vi "Initialize.vi"(8 "error in (no error)":errorcluster, 11 "AG in":refnum<class "AG.lvclass">) -> (0 "error out":errorcluster, 3 "AG out":refnum<class "AG.lvclass">)   [LabVIEW 2018, in "AG.lvclass"]
uses:
  AG.lvclass
  AG.lvclass/AG.ctl
  Client/Client.lvclass
  Comm/Stream/Stream.lvclass
  Log/Log.lvclass
  Device/angles/angles.lvclass
  StateMachine/State Machine.lvclass
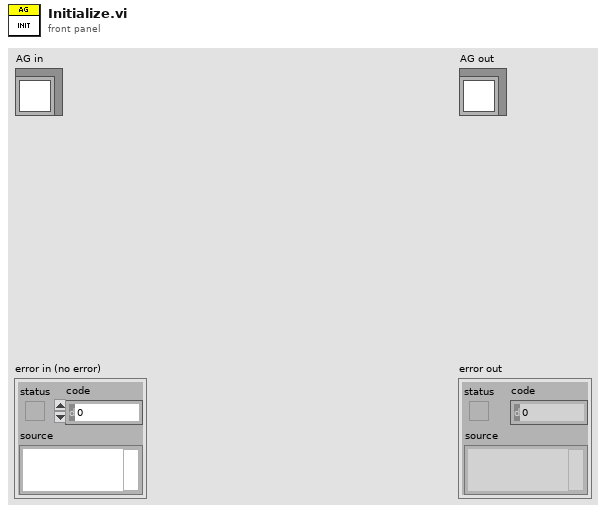
[diagram p1: front panel]
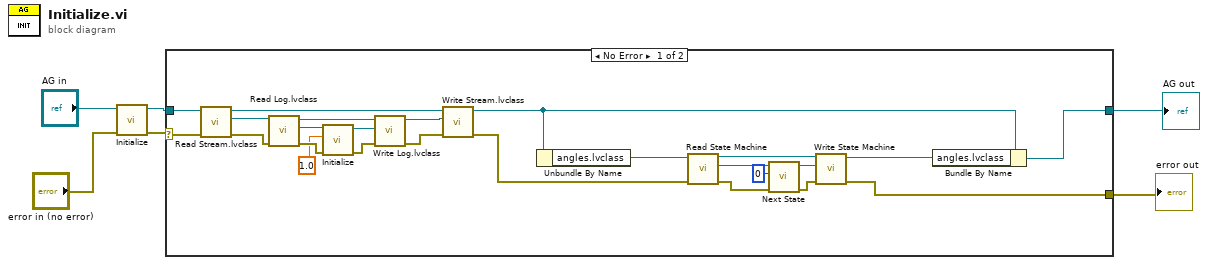
[diagram p0: block diagram]
diagram:
  n1 = call-parent "Initialize.vi"("error in (no error)"="error in (no error)", "Client in"="AG in") -> ("error out"=w3:errorcluster, "Client out"=w4:refnum<class "AG.lvclass">)  [unwired: 8 in]
  n2 = case shown="No Error" w3 {
    selector: w3 -> [w9 w33]
    tunnel: [w23 w32] -> w1
    tunnel: w4 -> [w10 w32]
    tunnel: [w11 w33] -> w2
    frame No Error {
      n3 = call-dynamic "Read Stream.lvclass.vi"("error in (no error)"=w9, "Client in"=w10) -> ("error out"=w7:errorcluster, "Stream.lvclass"=w8:refnum<class "Stream.lvclass">, "Client out"=w31:refnum<class "AG.lvclass">)  [unwired: 7 in]
      n4 = call-dynamic "Read Log.lvclass.vi"("error in (no error)"=w7, "Comm in"=w8) -> ("error out"=w19:errorcluster, "Log.lvclass"=w21:refnum<class "Log.lvclass">, "Comm out"=w22:refnum<class "Stream.lvclass">)  [unwired: 7 in]
      n5 = call-dynamic "Initialize.vi"("error in (no error)"=w19, "Level"=1.0, "Log in"=w21) -> ("error out"=w18:errorcluster, "Log out"=w20:refnum<class "Log.lvclass">)  [unwired: 7 in]
      n6 = call-dynamic "Write Log.lvclass.vi"("error in (no error)"=w18, "Log.lvclass"=w20, "Comm in"=w22) -> ("error out"=w16:errorcluster, "Comm out"=w17:refnum<class "Stream.lvclass">)  [unwired: 7 in]
      n7 = call-dynamic "Write Stream.lvclass.vi"("error in (no error)"=w16, "Stream.lvclass"=w17, "Client in"=w31) -> ("error out"=w13:errorcluster, "Client out"=w24:refnum<class "AG.lvclass">)  [unwired: 7 in]
      n8 = Unbundle By Name(w24) -> ("angles.lvclass"=w14:refnum<class "angles.lvclass">)
      n9 = call-dynamic "Read State Machine.vi"("error in (no error)"=w13, "Device in"=w14) -> ("error out"=w27:errorcluster, "State Machine.lvclass"=w30:refnum<class "State Machine.lvclass">, "Device out"=w29:refnum<class "angles.lvclass">)  [unwired: 7 in]
      n10 = call "Next State.vi"("error in (no error)"=w27, "New_State"=0, "State Machine in"=w30) -> ("error out"=w26:errorcluster, "State Machine out"=w28:refnum<class "State Machine.lvclass">)  [unwired: 7 in]
      n11 = call-dynamic "Write State Machine.vi"("error in (no error)"=w26, "State Machine.lvclass"=w28, "Device in"=w29) -> ("error out"=w11:errorcluster, "Device out"=w25:refnum<class "angles.lvclass">)  [unwired: 7 in]
      n12 = Bundle By Name(cluster=w24, "angles.lvclass"=w25) -> (w23:refnum<class "AG.lvclass">)
    }
    frame Error {
    }
  }
  "error out" <- w2
  "AG out" <- w1
